vi "setData.vi"(8 "error in (no error)":errorcluster, 10 "data":T1, 11 "reference in":refnum<class "subject.lvclass">) -> (0 "error out":errorcluster, 3 "reference out":refnum<class "subject.lvclass">)   [LabVIEW 2015, in "subject.lvclass"]
uses:
  subject.lvclass
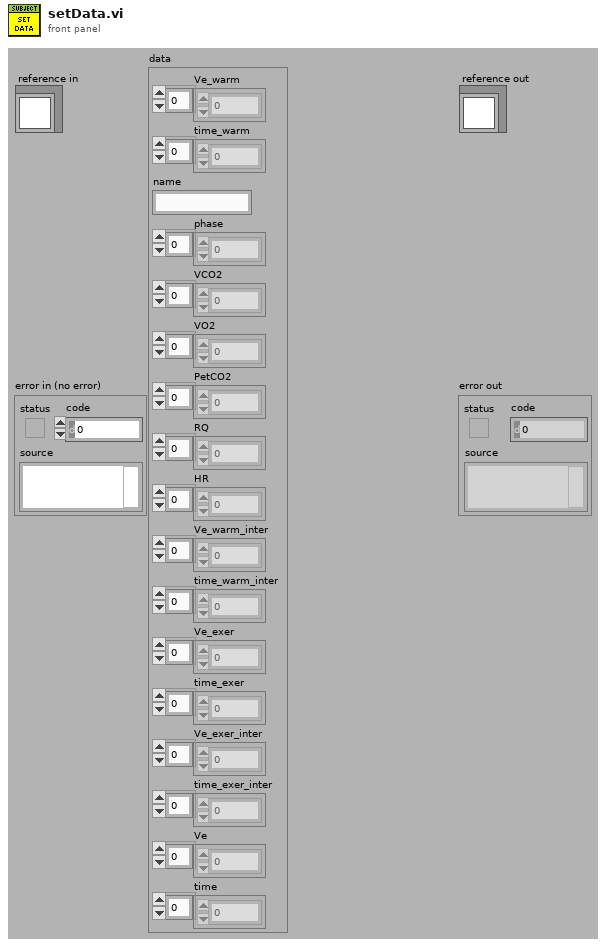
[diagram p1: front panel]
types:
  T1 = cluster{"Ve_warm":dbl[], "time_warm":dbl[], "name":string, "phase":dbl[], "VCO2":dbl[], "VO2":dbl[], "PetCO2":dbl[], "RQ":dbl[], "HR":dbl[], "Ve_warm_inter":dbl[], "time_warm_inter":dbl[], "Ve_exer":dbl[], "time_exer":dbl[], "Ve_exer_inter":dbl[], "time_exer_inter":dbl[], "Ve":dbl[], "time":dbl[]}
  T2 = typedef "subject.lvclass/ObjectAttributesRef.ctl" = refnum<data-value>
  T3 = typedef "subject.lvclass/ObjectAttributes.ctl" = cluster{"MyAttribute":dbl, "data":cluster{"Ve_warm":dbl[], "time_warm":dbl[], "name":string, "phase":dbl[], "VCO2":dbl[], "VO2":dbl[], "PetCO2":dbl[], "RQ":dbl[], "HR":dbl[], "Ve_warm_inter":dbl[], "time_warm_inter":dbl[], "Ve_exer":dbl[], "time_exer":dbl[], "Ve_exer_inter":dbl[], "time_exer_inter":dbl[], "Ve":dbl[], "time":dbl[]}, "results_5l":cluster{"EOV":bool, "osci_amplitude":dbl[], "osci_width":dbl[], "peak_location":dbl[]}, "results_15percent":cluster{"EOV":bool, "osci_amplitude":dbl[], "osci_width":dbl[], "peak_location":dbl[]}, "supportData":cluster{"peaksAmplitude":dbl[], "iPeaksLocation":dbl[], "valesAmplitude":dbl[], "iValesLocation":dbl[], "threshold":dbl, "width_warm":i32, "meanAmpl_warm":i32, "#_peaks":i32}}
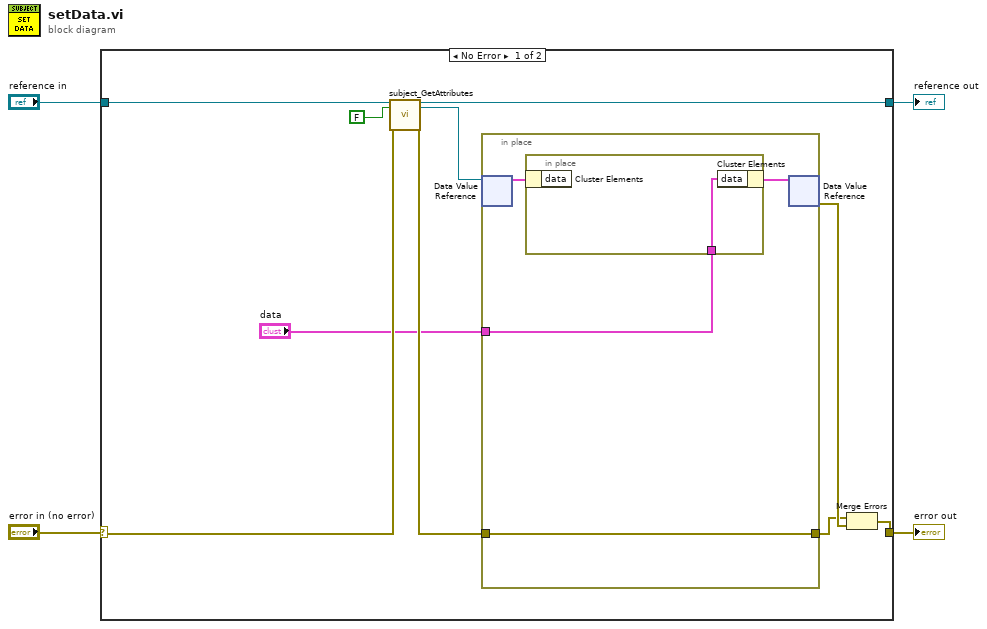
[diagram p0: block diagram]
diagram:
  n1 = case shown="No Error" "error in (no error)" {
    selector: "error in (no error)" -> [w9 w21]
    tunnel: [w14 w21] -> w3
    tunnel: [w7 w20] -> w1
    tunnel: "reference in" -> [w11 w20]
    frame No Error {
      n2 = call "subject_GetAttributes.vi"("reference in"=w11, "return data? (T)"=FALSE, "error in (no error)"=w9) -> ("reference out"=w7:refnum<class "subject.lvclass">, "attributes ref"=w6:T2, "error out"=w8:errorcluster)  [unwired: 13 in, 1 out]
      n3 = in-place {
        in-place-border: w8 -> [w16]
        in-place-border: [w16] -> w12
        in-place-border: "data" -> [w15]
        n4 = in-place-dvr #1(w6) -> (w17:T3)  [unwired: 1 out]
        n5 = in-place {
          in-place-border: w15 -> [w19]
          n6 = in-place-cluster #2(w17) -> ()  [unwired: 1 out]
          n7 = in-place-cluster #2("data"=w19) -> (w18:T3)
        }
        n8 = in-place-dvr #1(w18) -> (w13:errorcluster)  [unwired: 1 out]
      }
      n9 = Merge Errors(w12, w13) -> (w14:errorcluster)
    }
    frame Error {
    }
  }
  "error out" <- w3
  "reference out" <- w1
